vi "SerialDataReceive.vi"() -> ()   [LabVIEW 2019]
doc: "This example performs writes and reads on a serial port, as directed by the user. You can press the Write and Read buttons, and change the Read Count, while the example is running.\n\nThe parameters set for the serial port must match the parameters of the connected instrument or device. In this example, the Read Count parameter specifies the number of bytes that the serial port reads. If there were more bytes at the port than the specified number, those bytes would not be read. If there were less bytes at the port than the specified number, you would receive a timeout error.\n\nThis example expands upon the flow control options for XON and XOFF, allowing the user to choose those control characters. Also, the user can enable or disable a termination character. Some devices require a termination character in order to identify the end of command strings. Some devices send a termination character to signify the end of data to be read. This example shows how you can end the Read operation once a termination character is detected in the buffer and/or append a termination character at the end of the Write data."
uses:
  C:/Program Files/National Instruments/LabVIEW 2019/examples/Instrument IO/Serial/support/Serial - Settings.ctl
  <vilib>/Instr/_visa.llb/VISA Configure Serial Port (Instr).vi
panel:
  out "Details":string
  in  "Start SMS Send":bool
  in  "SMS Details":string="*IDN?"
  in  "Serial Settings":T1={"baud rate"=9600, "data bits"=8, "parity"=enum."None", "stop bits"=10, "flow control"=0} {"flow control" items=["None"=0, "XON/XOFF"=1, "RTS/CTS"=2, "DTR/DSR"=4]; "stop bits" items=["1.0"=10, "1.5"=15, "2.0"=20]; "data bits" min=5 max=8 step=1; "baud rate" items=["75"=75, "110"=110, "134"=134, "150"=150, "300"=300, "600"=600, "1200"=1200, "1800"=1800, "2400"=2400, "4800"=4800, "7200"=7200, "9600"=9600, "14400"=14400, "19200"=19200, "28800"=28800, "38400"=38400, "56000"=56000, "57600"=57600, "115200"=115200, "128000"=128000, "230400"=230400]}
  out "Heart Rate":dbl(knob) scale=0.0..150.0
  out "Thermometer":dbl(slide) scale=0.0..100.0
  out "ECG":dbl(graph)=-207.0
  out "Data 1D":dbl[](array[numeric]) caption="array" format="%#_2f"
  in  "Stop":bool
  in  "Read Count":u32=1000
  in  "Start Reading":bool
  in  "COM Port":refnum<visa-resource-name>="COM1"
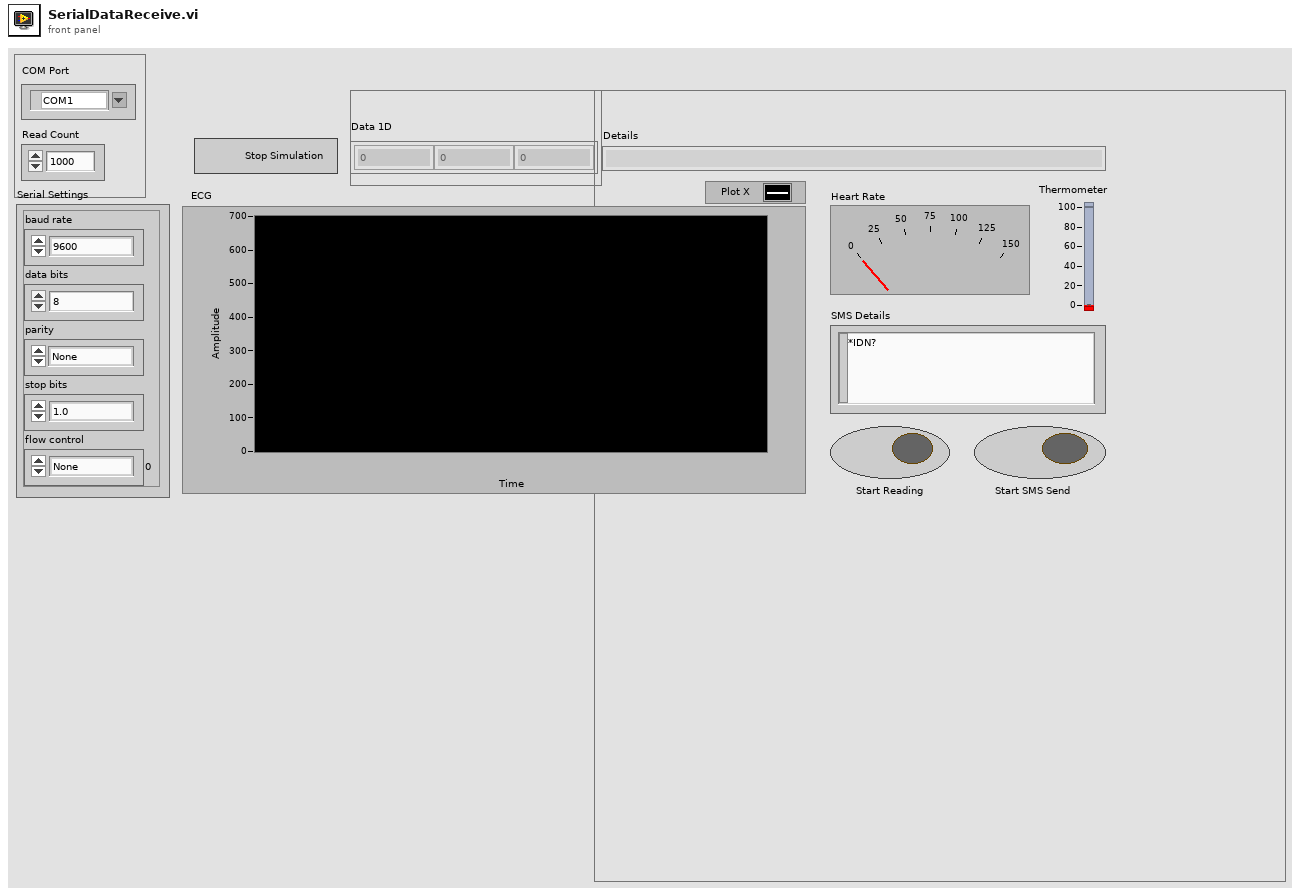
[diagram p1: front panel]
types:
  T1 = typedef "Serial - Settings.ctl" = cluster{"baud rate":u32, "data bits":u16, "parity":enum16{"None", "Odd", "Even", "Mark", "Space"}, "stop bits":u16, "flow control":u16}
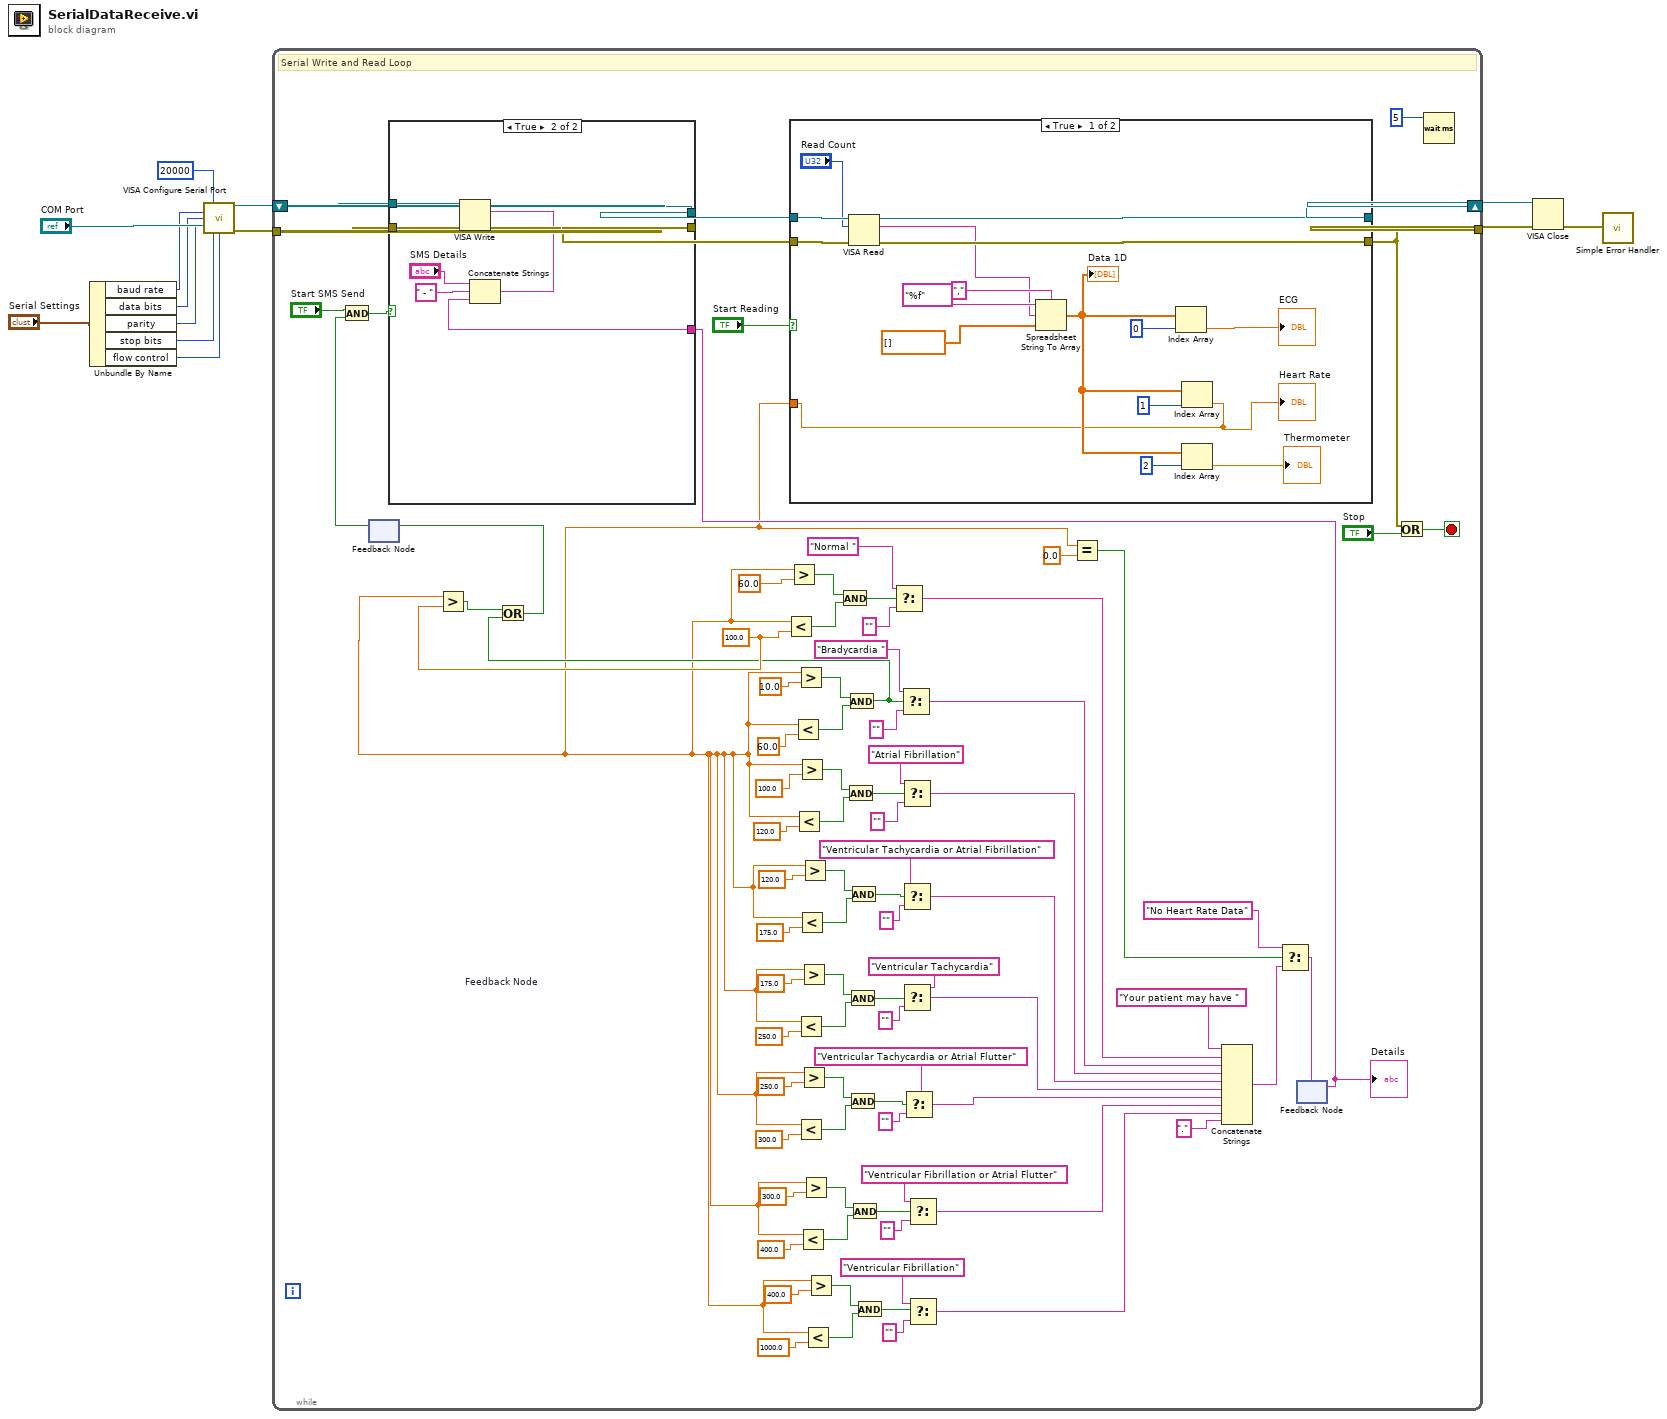
[diagram p0: block diagram]
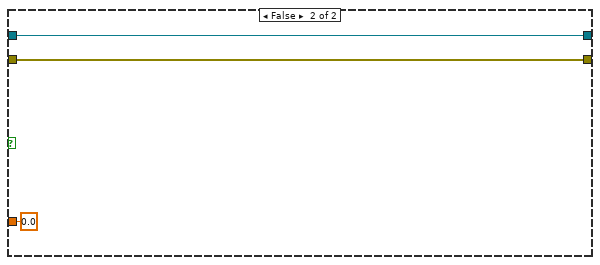
[diagram p3: hidden frame]
diagram:
  n1 = Unbundle By Name("Serial Settings") -> ("baud rate"=w6:u32, "data bits"=w5:u16, "parity"=w4:enum16{"None", "Odd", "Even", "Mark", "Space"}, "stop bits"=w3:u16, "flow control"=w2:u16)
  n2 = call-poly "VISA Configure Serial Port"("VISA resource name"="COM Port", "timeout (10sec)"=u32 20000, "baud rate (9600)"=w6, "data bits (8)"=w5, "parity (0:none)"=w4, "stop bits (10: 1 bit)"=w3, "flow control (0:none)"=w2) -> ("VISA resource name out"=w9:refnum<visa-resource-name>, "error out"=w8:errorcluster)  [unwired: 3 in, 4 out]
  n3 = while {
    shift-right: [w101] -> w10
    shift-left: w9 -> [w94]
    tunnel: w8 -> [w93]
    tunnel: [w100] -> w11
    stop <- w97 stop-if-true
    w24 = 100.0 ("y")
    # "Serial Write and Read Loop"
    n4 = feedback #1 "Feedback Node"() -> (w22:bool)  [unwired: 1 in]
    n5 = And(x="Start SMS Send", y=w22) -> (x .and. y?=w29:bool)
    n6 = feedback #2() -> (w21:string)  [unwired: 1 in]
    "Details" <- w21
    n7 = case shown="True" w29 {
      tunnel: w94 -> [w103 w111]
      tunnel: w93 -> [w102 w110]
      tunnel: [w103 w109] -> w96
      tunnel: [w102 w108] -> w95
      tunnel: w21 -> [_ w105]
      frame False {
      }
      frame True {
        n8 = Concatenate Strings("SMS Details", " - " ("string"), w105) -> (w106:string)
        n9 = VISA Write(VISA resource name=w111, write buffer=w106, error in (no error)=w110) -> (VISA resource name out=w109:refnum<visa-resource-name>, error out=w108:errorcluster)  [unwired: 1 out]
      }
    }
    n10 = case shown="True" "Start Reading" {
      tunnel: [w125 w130] -> w101
      tunnel: w96 -> [w127 w130]
      tunnel: [w123 w129] -> w100
      tunnel: w95 -> [w126 w129]
      tunnel: [w112 0.0 ("String")] -> w19
      frame True {
        n11 = VISA Read(VISA resource name=w127, byte count="Read Count", error in (no error)=w126) -> (VISA resource name out=w125:refnum<visa-resource-name>, read buffer=w119:string, error out=w123:errorcluster)  [unwired: 1 out]
        n12 = Spreadsheet String To Array(delimiter (Tab)=",", format string="%f", spreadsheet string=w119, array type (2D Dbl)=dbl[] [] ("Data Graph")) -> (array=w113:dbl[])
        "Data 1D" <- w113
        n13 = Index Array "Index Array"(array=w113, index=0 ("disabled index (col)")) -> (element=→"ECG":dbl)
        n14 = Index Array(array=w113, index=1 ("disabled index (col)")) -> (element=w112:dbl)
        "Heart Rate" <- w112
        n15 = Index Array(array=w113, index=2 ("disabled index (col)")) -> (element=→"Thermometer":dbl)
      }
      frame False {
      }
    }
    n16 = Greater?(x=w19, y=w24) -> (0:w28:bool)
    n17 = Less?(x=w19, y=w24) -> (x < y?=w39:bool)
    n18 = Greater?(x=w19, y=60.0) -> (0:w40:bool)
    n19 = Less?(x=w19, y=60.0) -> (x < y?=w43:bool)
    n20 = Less?(x=w19, y=120.0) -> (x < y?=w89:bool)
    n21 = Greater?(x=w19, y=10.0) -> (0:w44:bool)
    n22 = Less?(x=w19, y=250.0) -> (x < y?=w80:bool)
    n23 = Less?(x=w19, y=300.0) -> (x < y?=w76:bool)
    n24 = Greater?(x=w19, y=100.0) -> (0:w90:bool)
    n25 = Less?(x=w19, y=175.0) -> (x < y?=w84:bool)
    n26 = Less?(x=w19, y=400.0) -> (x < y?=w72:bool)
    n27 = Greater?(x=w19, y=175.0) -> (0:w81:bool)
    n28 = Greater?(x=w19, y=250.0) -> (0:w77:bool)
    n29 = Greater?(x=w19, y=120.0) -> (0:w85:bool)
    n30 = Greater?(x=w19, y=300.0) -> (0:w73:bool)
    n31 = Less?(x=w19, y=1000.0) -> (x < y?=w68:bool)
    n32 = Greater?(x=w19, y=400.0) -> (0:w69:bool)
    n33 = And(x=w40, y=w39) -> (x .and. y?=w38:bool)
    n34 = And(x=w90, y=w89) -> (x .and. y?=w88:bool)
    n35 = And(x=w44, y=w43) -> (x .and. y?=w20:bool)
    n36 = Or(x=w28, y=w20) -> (x .or. y?=w23:bool)
    n37 = feedback-in #1(w23) -> ()
    n38 = And(x=w81, y=w80) -> (x .and. y?=w64:bool)
    n39 = And(x=w77, y=w76) -> (x .and. y?=w65:bool)
    n40 = And(x=w85, y=w84) -> (x .and. y?=w63:bool)
    n41 = And(x=w73, y=w72) -> (x .and. y?=w66:bool)
    n42 = And(x=w69, y=w68) -> (x .and. y?=w67:bool)
    n43 = Select(t="Normal ", s=w38, f="") -> (s? t:f=w31:string)
    n44 = Select(t="Bradycardia ", s=w20, f="") -> (s? t:f=w32:string)
    n45 = Select(t="Atrial Fibrillation", s=w88, f="") -> (s? t:f=w33:string)
    n46 = Select(t="Ventricular Tachycardia or Atrial Fibrillation", s=w63, f="") -> (s? t:f=w34:string)
    n47 = Select(t="Ventricular Tachycardia", s=w64, f="") -> (s? t:f=w35:string)
    n48 = Select(t="Ventricular Tachycardia or Atrial Flutter", s=w65, f="") -> (s? t:f=w48:string)
    n49 = Select(t="Ventricular Fibrillation or Atrial Flutter", s=w66, f="") -> (s? t:f=w49:string)
    n50 = Select(t="Ventricular Fibrillation", s=w67, f="") -> (s? t:f=w47:string)
    n51 = Equal?(x=w19, y=0.0) -> (x = y?=w17:bool)
    n52 = Concatenate Strings "Concatenate Strings"("Your patient may have " ("string"), w31, w32, w33, w34, w35, w48, w49, w47, "." ("string")) -> (w16:string)
    n53 = Select(t="No Heart Rate Data", s=w17, f=w16) -> (s? t:f=w15:string)
    n54 = feedback-in #2(w15) -> ()
    n55 = Or(x=w100, y="Stop") -> (x .or. y?=w97:bool)
    n56 = Wait (ms)(milliseconds to wait=u32 5) -> ()  [unwired: 1 out]
  }
  n57 = VISA Close(VISA resource name=w10, error in (no error)=w11) -> (error out=w12:errorcluster)
  n58 = call <vilib>:"Simple Error Handler.vi"("error in (no error)"=w12) -> ()  [unwired: 1 in, 8 out]
